vi "Get Name.vi"(8 "error in (no error)":errorcluster, 11 "Item in":refnum<class "Item.lvclass">) -> (0 "error out":errorcluster, 2 "Name":string, 3 "Item out":refnum<class "Item.lvclass">)   [LabVIEW 2020, in "Item.lvclass"]
uses:
  Item.lvclass
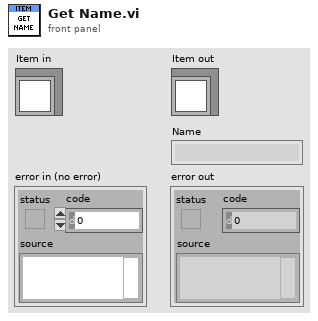
[diagram p1: front panel]
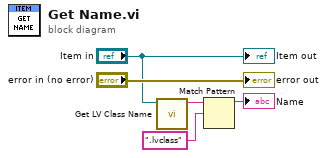
[diagram p0: block diagram]
diagram:
  n1 = call <vilib>:"Get LV Class Name.vi"("object"="Item in") -> ("class name"=w3:string)  [unwired: 9 in, 1 out]
  n2 = Match Pattern(string=w3, regular expression=".lvclass") -> (before substring=→"Name":string)  [unwired: 1 in, 3 out]
  "error out" <- "error in (no error)"
  "Item out" <- "Item in"
